vi "Pision Save.vi"(6 "计算值":cluster{"X":dbl, "Y":dbl, "Z":dbl, "U":dbl}[](array[cluster]), 9 "三点":dbl[][](array[numeric]), 10 "列":i32, 11 "行":i32) -> (3 "Value":string)   [LabVIEW 2011]
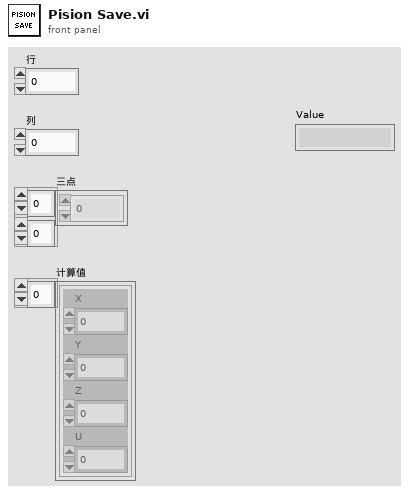
[diagram p1: front panel]
types:
  T1 = cluster{"X":string, "Y":string, "Z":string, "U":string}[]
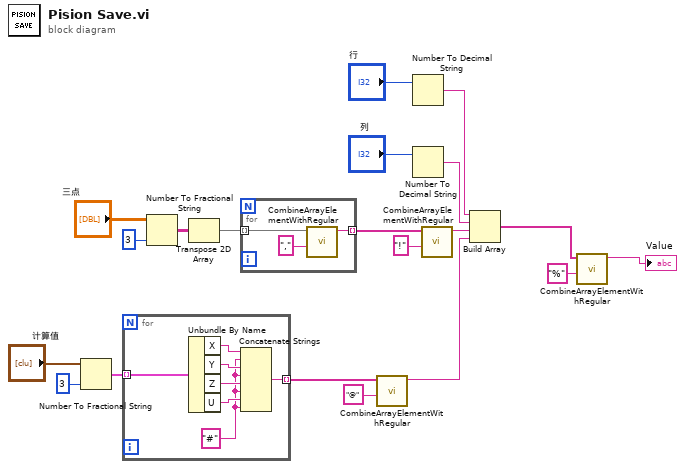
[diagram p0: block diagram]
diagram:
  n1 = Number To Fractional String(number="计算值", precision (6)=i16 3 ("精度(6)")) -> (F-format string=w14:T1)  [unwired: 2 in]
  n2 = for {
    tunnel: w14 -> [w27] mode=indexing
    tunnel: [w21] -> w15 mode=indexing
    w22 = "#" ("字符串")
    n3 = Unbundle By Name(w27) -> ("X"=w26:string, "Y"=w25:string, "Z"=w24:string, "U"=w23:string)
    n4 = Concatenate Strings(w26, w22, w25, w22, w24, w22, w23, w22) -> (w21:string)
  }
  n5 = Number To Fractional String(number="三点", precision (6)=i16 3 ("精度(6)")) -> (F-format string=w10:string[][])  [unwired: 2 in]
  n6 = Transpose 2D Array(2D array=w10) -> (transposed array=w11:string[][])
  n7 = for {
    tunnel: w11 -> [w30] mode=indexing
    tunnel: [w28] -> w13 mode=indexing
    n8 = call "CombineArrayElementWithRegular.vi"("regular expression"=",", "Array in"=w30) -> ("String out"=w28:string)  [unwired: 9 in]
  }
  n9 = call "CombineArrayElementWithRegular.vi"("regular expression"="@", "Array in"=w15) -> ("String out"=w20:string)  [unwired: 9 in]
  n10 = Number To Decimal String(number="行") -> (decimal integer string=w17:string)  [unwired: 1 in]
  n11 = Number To Decimal String(number="列") -> (decimal integer string=w18:string)  [unwired: 1 in]
  n12 = call "CombineArrayElementWithRegular.vi"("regular expression"="!", "Array in"=w13) -> ("String out"=w19:string)  [unwired: 9 in]
  n13 = Build Array(w17, w18, w19, w20) -> (w2:string[])
  n14 = call "CombineArrayElementWithRegular.vi"("regular expression"="%", "Array in"=w2) -> ("String out"=→"Value":string)  [unwired: 9 in]
